vi "insert impulse into waveform.vi"() -> ()   [LabVIEW 2020]
uses:
  <vilib>/Analysis/NI_AALBase.lvlib
panel:
  in  "timestamp":timestamp
  out "Waveform Graph":waveform(dbl)(graph)
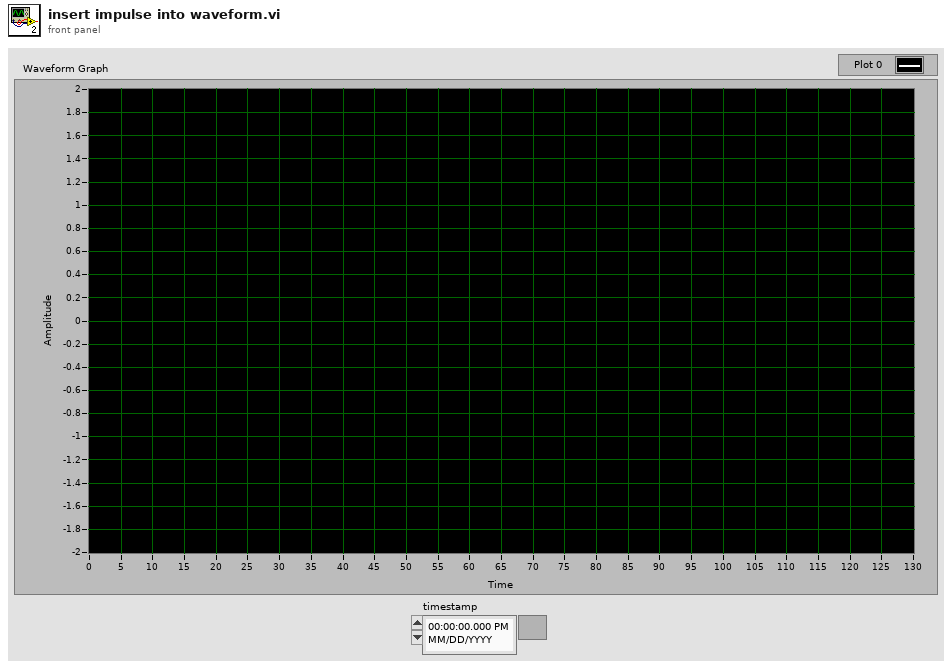
[diagram p1: front panel]
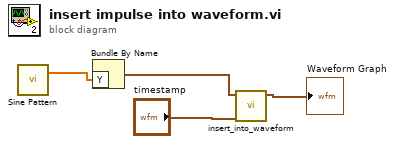
[diagram p0: block diagram]
diagram:
  n1 = call <vilib>:"Sine Pattern.vi"() -> ("Sinusoidal Pattern"=w4:dbl[])  [unwired: 4 in, 1 out]
  n2 = Bundle By Name("Y"=w4) -> (w3:waveform(dbl))  [unwired: 1 in]
  n3 = call "insert_into_waveform.vi"("timestamp"="timestamp", "waveform"=w3) -> ("updated waveform"=→"Waveform Graph":waveform(dbl))  [unwired: 9 in]
